vi "led_player_run.vi"(8 "error in (no error)":errorcluster, 10 "volume":i32, 11 "Refnum in":refnum<k21>) -> (1 "error out":errorcluster, 2 "Array":bool[](array[boolean]), 3 "Refnum out":refnum<k21>)   [LabVIEW 2022 SP3]
uses:
  <vilib>/DAQmx/miscellaneous.llb/DAQmx Fill In Error Info.vi
  <vilib>/DAQmx/write.llb/DAQmx Write (Digital 1D Bool 1Chan 1Samp).vi
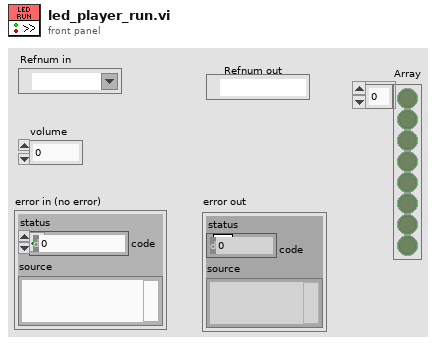
[diagram p1: front panel]
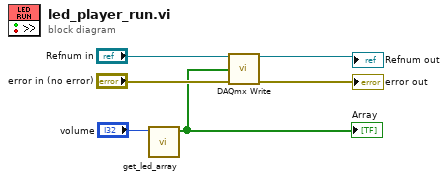
[diagram p0: block diagram]
diagram:
  n1 = call "get_led_array.vi"("y"="volume") -> ("Array"=w2:bool[])  [unwired: 10 in]
  "Array" <- w2
  n2 = call-poly <vilib>:"DAQmx Write.vi"("task/channels in"="Refnum in", "data"=w2, "error in"="error in (no error)") -> ("task out"=→"Refnum out":refnum<k21>, "error out"=→"error out":errorcluster)  [unwired: 10 in, 1 out]
